vi "RSZVB Get B Wave Receiver Power Calibration State.vi"(8 "error in (no error)":errorcluster {"code" format="%.0x"}, 9 "Port Number (1)":i32=1, 10 "Channel (1)":i32=1, 11 "VISA session":refnum<visa-resource-name>) -> (0 "error out":errorcluster {"code" format="%.0x"}, 2 "Receiver Power Calibration":bool, 3 "dup VISA session":refnum<visa-resource-name>)   [LabVIEW 2011]
doc: "This VI returns the state of the receiver power calibration for channel <Ch> and for the received waves Bn. \n\nRemote-control command(s):\n[SENSe<Ch>:]CORRection:POWer<port_no>[:STATe]?"
uses:
  _utility/RSZVB Global Data.vi
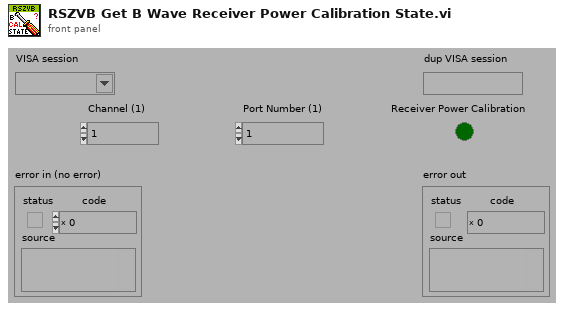
[diagram p1: front panel]
types:
  T1 = cluster{"Error Checking (T: On)":bool, "Installed Options":string[], "Data Valid?":bool, "Ports":i32, "Model":string[], "Option Checking (T: On)":bool}[]
  T2 = cluster{"Error Checking (T: On)":bool, "Installed Options":string[], "Data Valid?":bool, "Ports":i32, "Model":string[], "Option Checking (T: On)":bool}
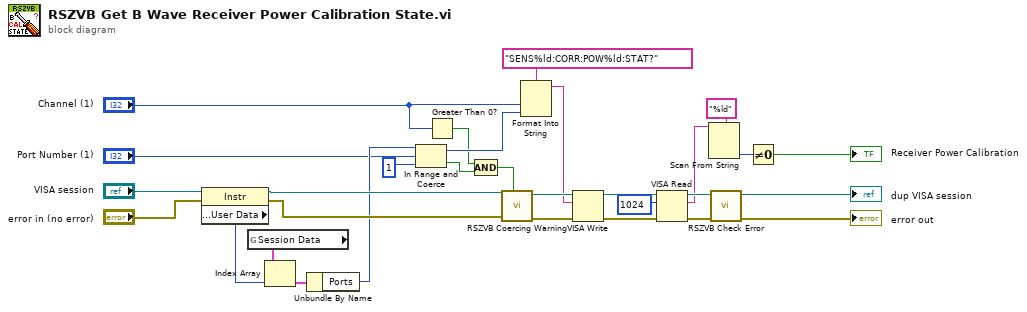
[diagram p0: block diagram]
diagram:
  n1 = property class="Instr"(reference="VISA session", error in="error in (no error)") -> (reference out=w15:refnum<visa-resource-name>, error out=w14:errorcluster, "General Settings:User Data"=w16:u32)
  n2 = global read "RSZVB Global Data.vi" "Session Data"() -> (w17:T1)
  n3 = Index Array(array=w17, index=w16) -> (element=w18:T2)
  n4 = Unbundle By Name(w18) -> ("Ports"=w11:i32)
  n5 = In Range and Coerce(upper limit=w11, x="Port Number (1)", lower limit=1) -> (coerced(x)=w10:i32, In Range?=w12:bool)
  n6 = Greater Than 0?(x="Channel (1)") -> (x > 0?=w9:bool)
  n7 = Compound Arithmetic op=AND(w9, w12) -> (w8:bool)
  n8 = call "RSZVB Coercing Warning.vi"("In Range?"=w8, "error in (no error)"=w14, "VISA session"=w15) -> ("error out"=w28:errorcluster, "dup VISA session"=w29:refnum<visa-resource-name>)  [unwired: 7 in]
  n9 = Format Into String(format string="SENS%ld:CORR:POW%ld:STAT?", "Channel (1)", w10) -> (resulting string=w27:string)  [unwired: 2 in, 1 out]
  n10 = VISA Write(VISA resource name=w29, write buffer=w27, error in (no error)=w28) -> (VISA resource name out=w20:refnum<visa-resource-name>, error out=w19:errorcluster)  [unwired: 1 out]
  n11 = VISA Read(VISA resource name=w20, byte count=u32 1024 ("byte count (0)"), error in (no error)=w19) -> (VISA resource name out=w25:refnum<visa-resource-name>, read buffer=w22:string, error out=w24:errorcluster)  [unwired: 1 out]
  n12 = Scan From String(format string="%ld", input string=w22) -> (output 1=w21:i32)  [unwired: 3 in, 3 out]
  n13 = call "RSZVB Check Error.vi"("error in (no error)"=w24, "VISA session"=w25) -> ("error out"=→"error out":errorcluster, "dup VISA session"=→"dup VISA session":refnum<visa-resource-name>)  [unwired: 8 in]
  n14 = Not Equal To 0?(x=w21) -> (x != 0?=→"Receiver Power Calibration":bool)
